vi "esdaq_analogWrite.vi"(2 "esdaqErrorInp":errorcluster, 3 "Value":u16, 4 "Channel":u8, 5 "esdaqPortInp":refnum<visa-resource-name>) -> (0 "esdaqErrorOut":errorcluster, 1 "esdaqPortOut":refnum<visa-resource-name>)   [LabVIEW 2019]
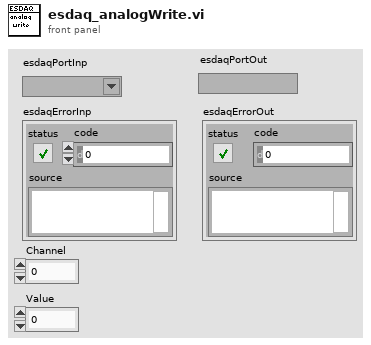
[diagram p1: front panel]
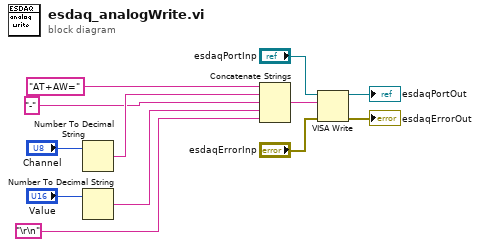
[diagram p0: block diagram]
diagram:
  n1 = Number To Decimal String(number="Channel") -> (decimal integer string=w9:string)  [unwired: 1 in]
  n2 = Number To Decimal String(number="Value") -> (decimal integer string=w7:string)  [unwired: 1 in]
  n3 = Concatenate Strings("AT+AW=", w9, "-", w7, "\r\n") -> (w5:string)
  n4 = VISA Write(VISA resource name="esdaqPortInp", write buffer=w5, error in (no error)="esdaqErrorInp") -> (VISA resource name out=→"esdaqPortOut":refnum<visa-resource-name>, error out=→"esdaqErrorOut":errorcluster)  [unwired: 1 out]
